vi "Second Order Step Response.vi"(8 "Error In":errorcluster, 9 "Time [s]":dbl[](array[numeric]), 10 "w0":dbl, 11 "xi":dbl) -> (0 "Error Out":errorcluster, 1 "Response":dbl[](array[numeric]))   [LabVIEW 2021]
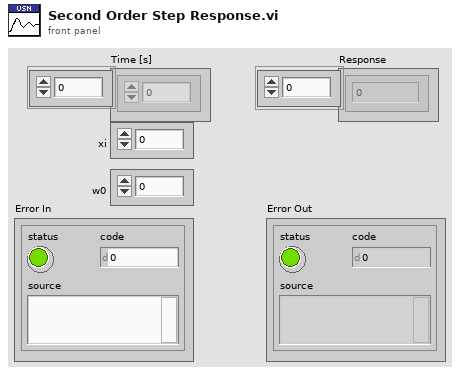
[diagram p1: front panel]
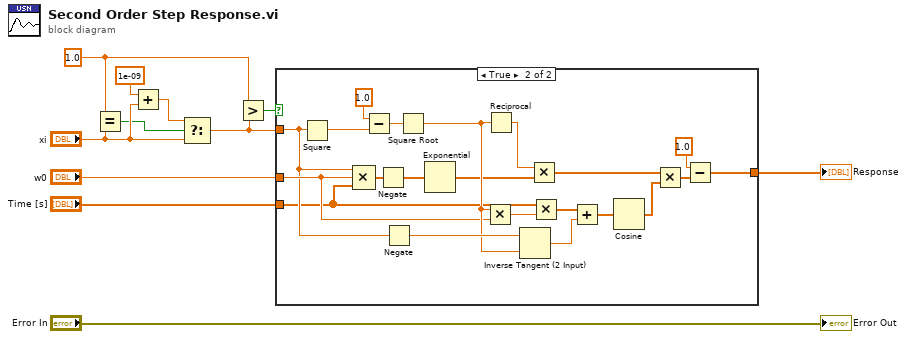
[diagram p0: block diagram]
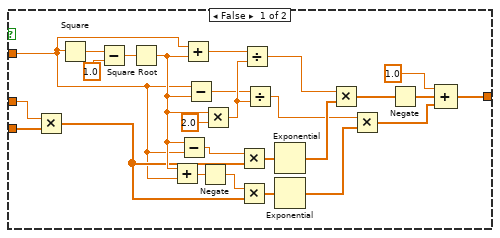
[diagram p2: hidden frame]
diagram:
  w7 = 1.0 ("y")
  n1 = Equal?(x=w7, y="xi") -> (x = y?=w2:bool)
  n2 = Add(x=1e-09, y="xi") -> (x+y=w4:dbl)
  n3 = Select(t=w4, s=w2, f="xi") -> (s? t:f=w1:dbl)
  n4 = Greater?(x=w7, y=w1) -> (0:w6:bool)
  n5 = case shown="True" w6 {
    tunnel: [w18 w47] -> w11
    tunnel: "w0" -> [w14 w41]
    tunnel: "Time [s]" -> [w15 w38]
    tunnel: w1 -> [w12 w40]
    frame False {
      n6 = Multiply(x=w14, y=w15) -> (x*y=w17:dbl[])
      n7 = Square(x=w12) -> (x^2=w24:dbl)
      n8 = Subtract(x=w24, y=1.0 ("x")) -> (x-y=w25:dbl)
      n9 = Square Root(x=w25) -> (sqrt(x)=w30:dbl)
      n10 = Add(x=w30, y=w12) -> (x+y=w28:dbl)
      n11 = Subtract(x=w30, y=w12) -> (x-y=w26:dbl)
      n12 = Add(x=w12, y=w30) -> (x+y=w23:dbl)
      n13 = Subtract(x=w12, y=w30) -> (x-y=w31:dbl)
      n14 = Negate(x=w28) -> (-x=w29:dbl)
      n15 = Multiply(x=w30, y=2.0) -> (x*y=w32:dbl)
      n16 = Multiply(x=w26, y=w17) -> (x*y=w27:dbl[])
      n17 = Multiply(x=w29, y=w17) -> (x*y=w16:dbl[])
      n18 = Divide(x=w23, y=w32) -> (x/y=w33:dbl)
      n19 = Divide(x=w31, y=w32) -> (x/y=w13:dbl)
      n20 = Exponential(1:w27) -> (0:w34:dbl[])
      n21 = Exponential(1:w16) -> (0:w35:dbl[])
      n22 = Multiply(x=w33, y=w34) -> (x*y=w19:dbl[])
      n23 = Multiply(x=w13, y=w35) -> (x*y=w37:dbl[])
      n24 = Negate(x=w19) -> (-x=w36:dbl[])
      n25 = Compound Arithmetic op=ADD(1.0 ("x"), w36, w37) -> (w18:dbl[])
    }
    frame True {
      n26 = Square(x=w40) -> (x^2=w56:dbl)
      n27 = Compound Arithmetic op=MULTIPLY(w40, w41, w38) -> (w57:dbl[])
      n28 = Subtract(x=1.0, y=w56) -> (x-y=w42:dbl)
      n29 = Negate(x=w57) -> (-x=w58:dbl[])
      n30 = Negate(x=w40) -> (-x=w46:dbl)
      n31 = Square Root(x=w42) -> (sqrt(x)=w45:dbl)
      n32 = Exponential(1:w58) -> (0:w39:dbl[])
      n33 = Multiply(x=w45, y=w41) -> (x*y=w53:dbl)
      n34 = Reciprocal(x=w45) -> (1/x=w54:dbl)
      n35 = Inverse Tangent (2 Input)(1:w45, 2:w46) -> (0:w43:dbl)
      n36 = Multiply(x=w54, y=w39) -> (x*y=w50:dbl[])
      n37 = Multiply(x=w38, y=w53) -> (x*y=w52:dbl[])
      n38 = Add(x=w52, y=w43) -> (x+y=w51:dbl[])
      n39 = Cosine(x=w51) -> (cos(x)=w44:dbl[])
      n40 = Multiply(x=w50, y=w44) -> (x*y=w49:dbl[])
      n41 = Subtract(x=1.0, y=w49) -> (x-y=w47:dbl[])
    }
  }
  "Response" <- w11
  "Error Out" <- "Error In"
